vi "relWaypoint.vi"(7 "Base Point":enum16{"Port", "Midpoint", "Starboard"}(ring), 8 "Error In":errorcluster, 9 "Y coord":i32, 10 "X coord":i32, 11 "PassBouy.lvclass":refnum<class "PassBouy.lvclass">) -> (0 "Error Out":errorcluster, 2 "UTM Location 3":T1 {"North" format="%#_10f"; "East" format="%#_8f"}, 3 "PassBouy.lvclass out":refnum<class "PassBouy.lvclass">)   [LabVIEW 2012, in "PassBouy.lvclass"]
uses:
  PassBouy.lvclass
  Data/TypeDefs/UTM Location.ctl
  <vilib>/Analysis/Matrix/Datatypes/RealMatrix.ctl
  PassBouy.lvclass/PassBouy.ctl
  <vilib>/Analysis/baseanly.llb/Unit Vector (DBL).vi
  <vilib>/Analysis/Matrix/Numeric/Conversions/Array To Matrix - RA.vi
  <vilib>/Analysis/Matrix/Numeric/Multiply/Multiply - RM,R.vi
  <vilib>/Analysis/Matrix/Numeric/Conversions/Matrix To Array - RM.vi
  <vilib>/Analysis/Matrix/Numeric/Multiply/Multiply - RM,RM.vi
  Waypoint/Waypoint.lvclass
  <vilib>/Analysis/NI_AALBase.lvlib
  <vilib>/Analysis/Matrix/NI_Matrix.lvlib
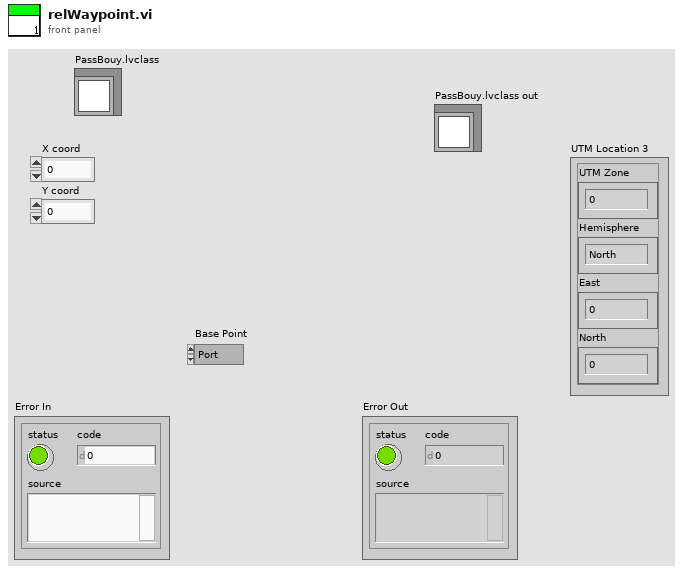
[diagram p1: front panel]
types:
  T1 = typedef "UTM Location.ctl" = cluster{"UTM Zone":dbl, "Hemisphere":enum16{"North", "South"}, "East":dbl, "North":dbl}
  T2 = typedef "NI_Matrix.lvlib/RealMatrix.ctl" = dbl[][]
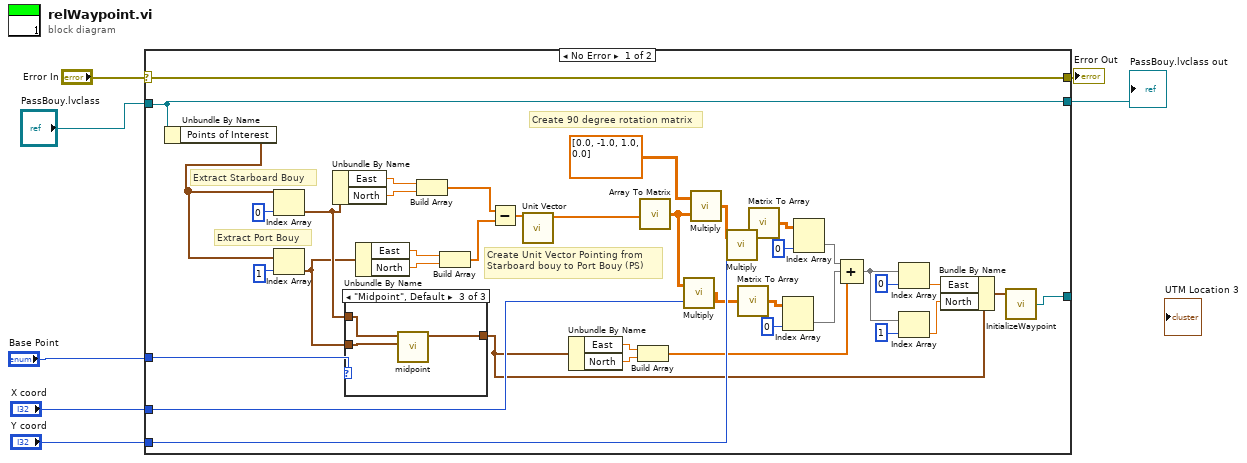
[diagram p0: block diagram]
diagram:
  n1 = case shown="No Error" "Error In" {
    selector: "Error In" -> [w47 w53]
    tunnel: [w47 w53] -> w5
    tunnel: "PassBouy.lvclass" -> [w46 w54]
    tunnel: [w46 w54] -> w6
    tunnel: "X coord" -> [w30 _]
    tunnel: "Y coord" -> [w28 _]
    tunnel: "Base Point" -> [w39 _]
    tunnel: [w15 _] -> _
    frame No Error {
      # "Create 90 degree rotation matrix"
      # "Create Unit Vector Pointing from\nStarboard bouy to Port Bouy (PS)"
      # "Extract Port Bouy"
      # "Extract Starboard Bouy"
      n2 = Unbundle By Name(w46) -> ("Points of Interest"=w43:T1[])
      n3 = Index Array(array=w43, index=0) -> (element=w42:T1)
      n4 = Index Array(array=w43, index=1) -> (element=w36:T1)
      n5 = Unbundle By Name(w42) -> ("East"=w41:dbl, "North"=w40:dbl)
      n6 = case shown="\"Midpoint\", Default" w39 {
        tunnel: w42 -> [w48 _ w52]
        tunnel: w36 -> [_ w49 w51]
        tunnel: [w48 w49 w50] -> w14
        frame "Starboard" {
        }
        frame "Port" {
        }
        frame "Midpoint", Default {
          n7 = call "midpoint.vi"("UTM Location 2"=w51, "UTM Location"=w52) -> ("UTM Location 3"=w50:T1)  [unwired: 8 in, 1 out]
        }
      }
      n8 = Unbundle By Name(w36) -> ("East"=w37:dbl, "North"=w38:dbl)
      n9 = Build Array(w41, w40) -> (w35:dbl[])
      n10 = Build Array(w37, w38) -> (w34:dbl[])
      n11 = Subtract(x=w35, y=w34) -> (x-y=w33:dbl[])
      n12 = call-poly <vilib>:"Unit Vector.vi"("Input Vector"=w33) -> ("Unit Vector"=w32:dbl[])  [unwired: 8 in, 2 out]
      n13 = Unbundle By Name(w14) -> ("East"=w27:dbl, "North"=w26:dbl)
      n14 = Build Array(w27, w26) -> (w21:dbl[])
      n15 = call-poly <vilib>:"Array To Matrix.vi"("Real 1D Array"=w32) -> ("Real Matrix (Column Vector)"=w31:T2)
      n16 = call-poly <vilib>:"Multiply.vi"("Real Scalar c"=w30, "Real Matrix A"=w31) -> ("A * c"=w24:T2)
      n17 = call-poly <vilib>:"Multiply.vi"("Real Matrix B"=w31, "Real Matrix A"=T2 [[0.0, -1.0], [1.0, 0.0]] ("matrix")) -> ("A * B"=w29:T2)
      n18 = call-poly <vilib>:"Multiply.vi"("Real Scalar c"=w28, "Real Matrix A"=w29) -> ("A * c"=w16:T2)
      n19 = call-poly <vilib>:"Matrix To Array.vi"("Real Matrix"=w24) -> ("Real 2D Array"=w23:dbl[][])
      n20 = call-poly <vilib>:"Matrix To Array.vi"("Real Matrix"=w16) -> ("Real 2D Array"=w18:dbl[][])
      n21 = Index Array(array=w23, index (col)=0 ("disabled index (col)")) -> (element=w20:dbl[])  [unwired: 1 in]
      n22 = Index Array(array=w18, index (col)=0 ("disabled index (col)")) -> (element=w17:dbl[])  [unwired: 1 in]
      n23 = Compound Arithmetic op=ADD(w17, w20, w21) -> (w9:dbl[])
      n24 = Index Array(array=w9, index=0) -> (element=w11:dbl)
      n25 = Index Array(array=w9, index=1) -> (element=w8:dbl)
      n26 = Bundle By Name(cluster=w14, "East"=w11, "North"=w8) -> (w13:T1)
      n27 = call "InitializeWaypoint.vi"("Coords"=w13) -> ("Waypoint Out"=w15:refnum<class "Waypoint.lvclass">)  [unwired: 2 in]
    }
    frame Error {
    }
  }
  "Error Out" <- w5
  "PassBouy.lvclass out" <- w6
